vi "Win32 Decode Img Stream.vi"(8 "error in (no error)":errorcluster, 10 "Dest Format":string(combo)="{d98c6b95-3efe-47d6-bb25-eb1748ab0cf1}", 11 "Image Data":u8[](array[numeric])) -> (0 "error out":errorcluster, 1 "Image Height":u32, 2 "Image Width":u32, 3 "Dest":u32[][](array[numeric]), 4 "Image Stride":u32)   [LabVIEW 2020]
uses:
  ole32.dll
  windowscodecs.dll
  shlwapi.dll
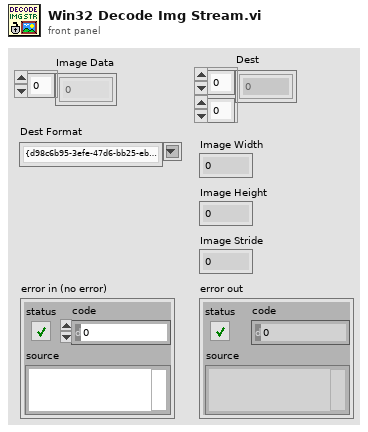
[diagram p1: front panel]
types:
  T1 = cluster{"GUID1":u32, "GUID2":u16, "GUID3":u16, "GUID4":cluster{"GUID4[0]":u8, "GUID4[1]":u8, "GUID4[2]":u8, "GUID4[3]":u8, "GUID4[4]":u8, "GUID4[5]":u8, "GUID4[6]":u8, "GUID4[7]":u8}}
  T2 = enum32{"Custom", "MedianCut", "FixedBW", "FixedHalftone8", "FixedHalftone27", "FixedHalftone64", "FixedHalftone125", "FixedHalftone216 / FixedWebPalette", "FixedHalftone252", "FixedHalftone256", "FixedGray4", "FixedGray16", "FixedGray256"}
  T3 = enum32{"None / Solid", "Ordered4x4", "Ordered8x8", "Ordered16x16", "Spiral4x4", "Spiral8x8", "DualSpiral4x4", "DualSpiral8x8", "ErrorDiffusion"}
  T4 = enum32{"NoCache", "CacheOnDemand", "CacheOnLoad"}
  T5 = cluster{"puiWidth":u32, "puiWidth":u32, "puiWidth":u32, "puiHeight":u32}
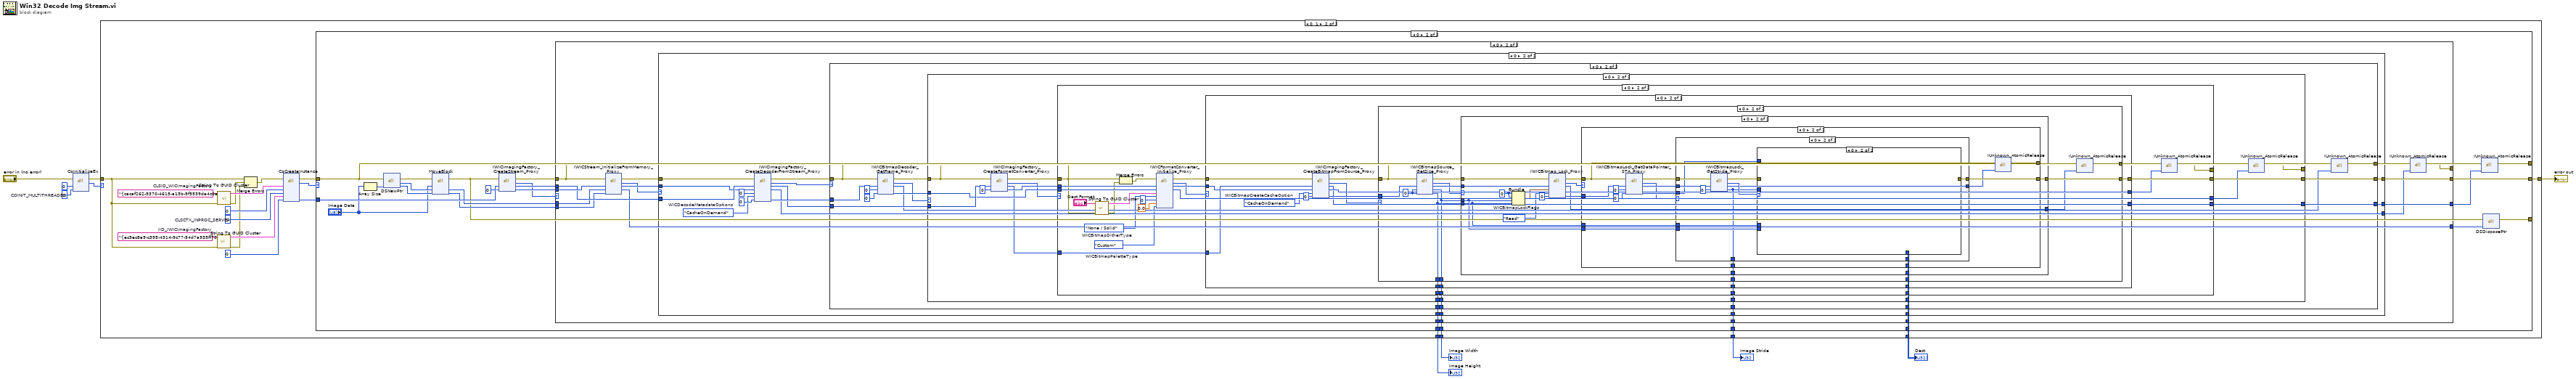
[diagram p0: block diagram]
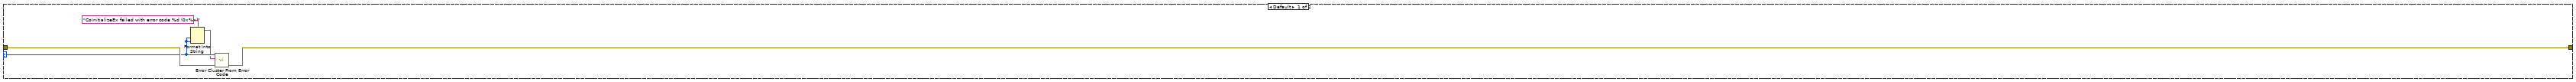
[diagram p2: hidden frame]
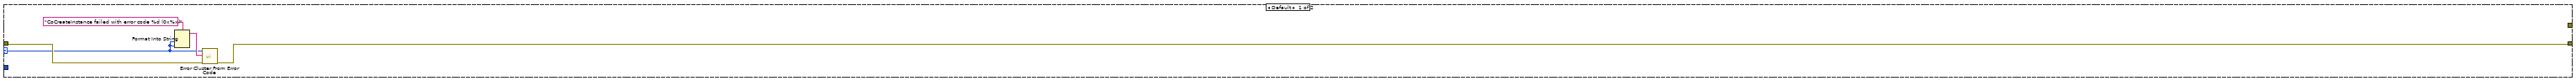
[diagram p3: hidden frame]
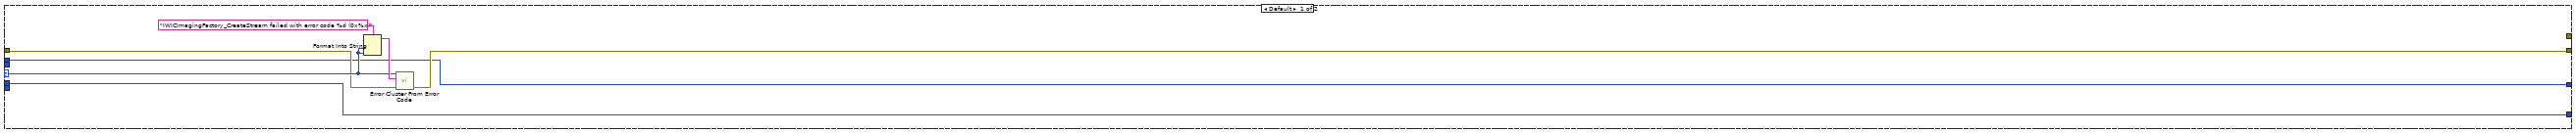
[diagram p4: hidden frame]
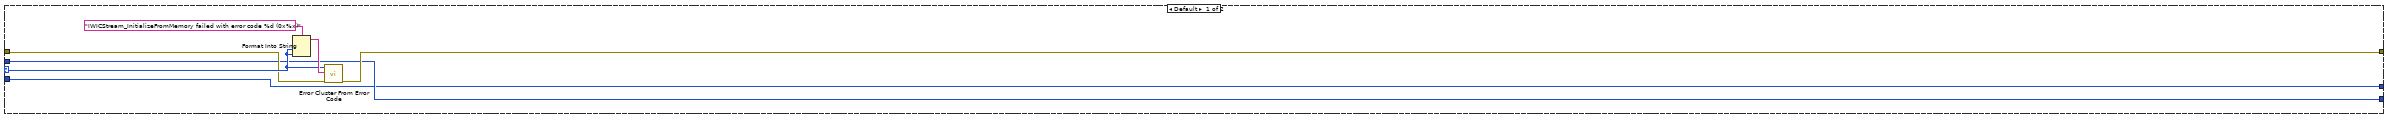
[diagram p5: hidden frame]
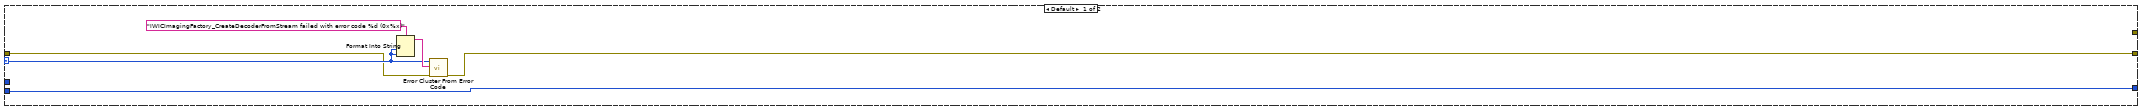
[diagram p6: hidden frame]
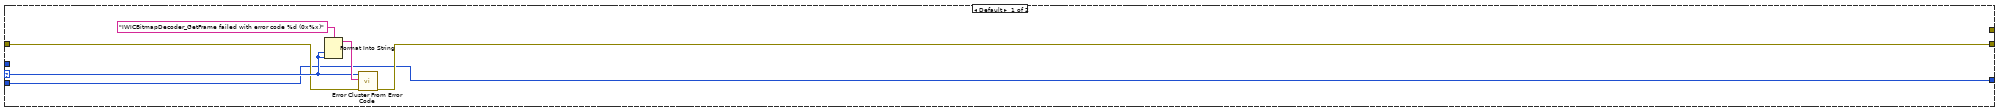
[diagram p7: hidden frame]
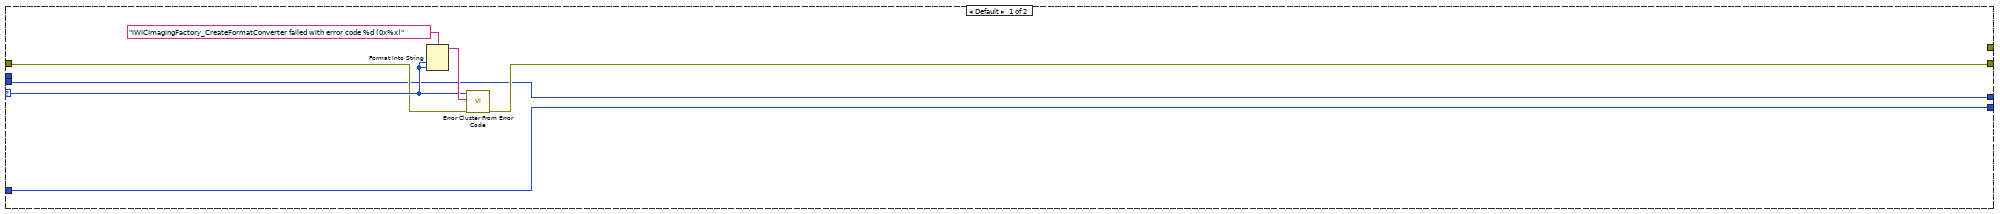
[diagram p8: hidden frame]
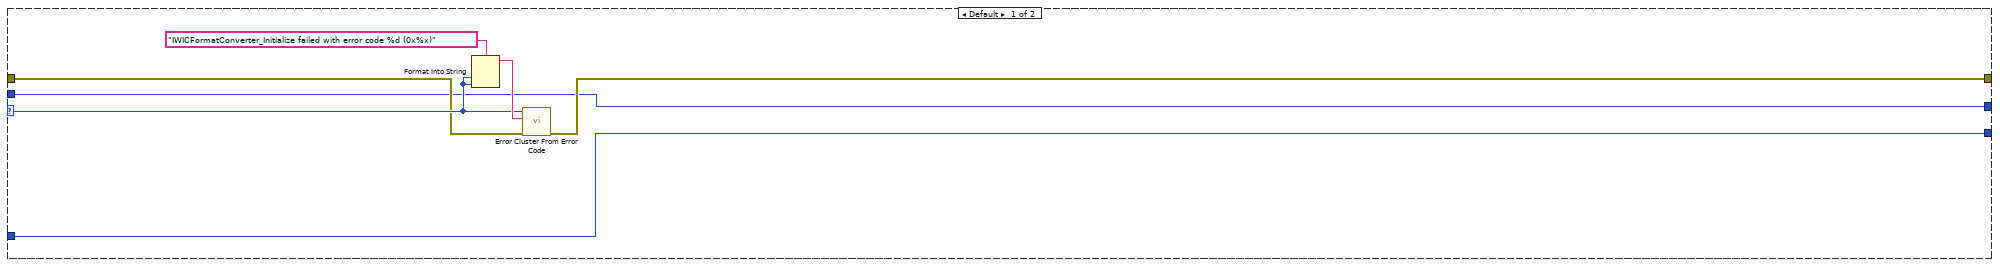
[diagram p9: hidden frame]
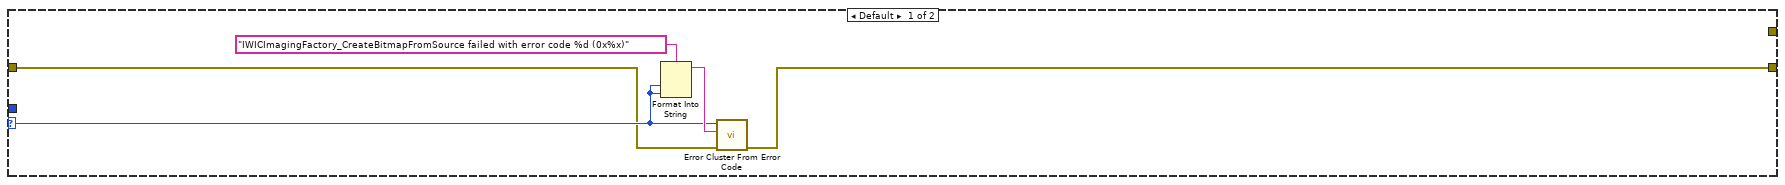
[diagram p10: hidden frame]
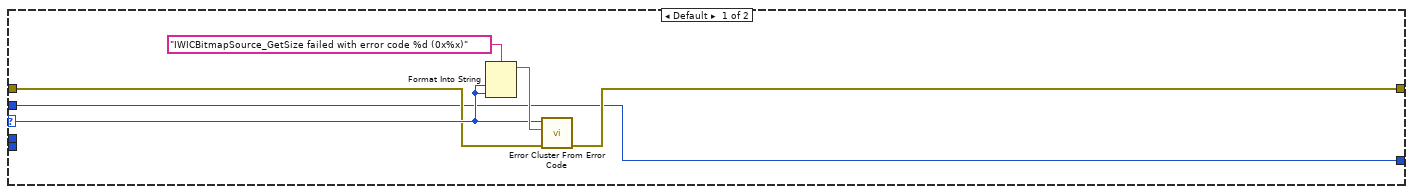
[diagram p11: hidden frame]
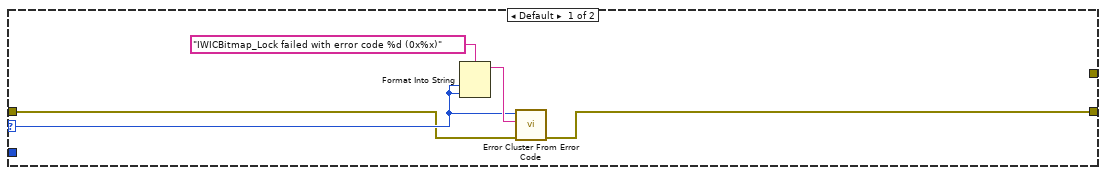
[diagram p12: hidden frame]
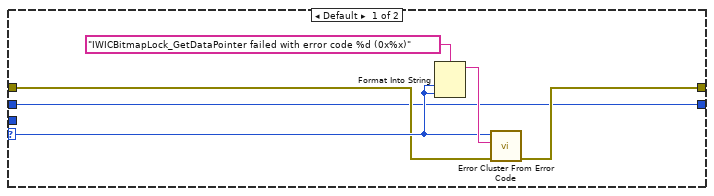
[diagram p13: hidden frame]
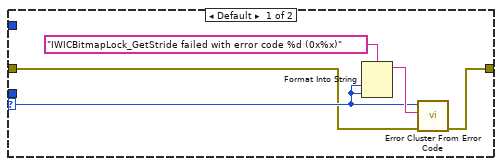
[diagram p14: hidden frame]
diagram:
  w9 = u32 0  # COINIT_MULTITHREADED
  n1 = dll-call lib="ole32.dll" fn="CoInitializeEx"(error in="error in (no error)", "pvReserved"=u64 0, "dwCoInit"=w9) -> (error out=w8:errorcluster, "Return"=w6:i32)  [unwired: 4 in, 1 out]
  n2 = case shown="0, 1" w6 {
    selector: w6 -> [w13 _]
    tunnel: w8 -> [w15 w25]
    tunnel: [w11 w20] -> w5
    tunnel: [_ w19] -> w4
    tunnel: [_ w18] -> w3
    tunnel: [_ w17] -> w2
    tunnel: [_ w16] -> w1
    frame Default {
      n3 = Format Into String(format string="CoInitializeEx failed with error code %d (0x%x)" ("error message (\"\")"), w13, w13) -> (resulting string=w12:string)  [unwired: 2 in, 1 out]
      n4 = call <vilib>:"Error Cluster From Error Code.vi"("error in (no error)"=w15, "error message (\"\")"=w12, "error code (0)"=w13) -> ("error out"=w11:errorcluster)  [unwired: 6 in]
    }
    frame 0, 1 {
      w30 = "{ec5ec8a9-c395-4314-9c77-54d7a935ff70}"  # IID_IWICImagingFactory
      w32 = u32 1  # CLSCTX_INPROC_SERVER
      w34 = "{cacaf262-9370-4615-a13b-9f5539da4c0a}"  # CLSID_WICImagingFactory
      n5 = call "String To GUID Cluster.vi"("error in (no error)"=w25, "Input String"=w30) -> ("error out"=w23:errorcluster, "GUID"=w29:T1)  [unwired: 4 in]
      n6 = call "String To GUID Cluster.vi"("error in (no error)"=w25, "Input String"=w34) -> ("error out"=w24:errorcluster, "GUID"=w33:T1)  [unwired: 4 in]
      n7 = Merge Errors(w25, w24, w23) -> (w22:errorcluster)
      n8 = dll-call lib="ole32.dll" fn="CoCreateInstance"(error in=w22, "rclsid"=w33, "pUnkOuter"=u64 0, "dwClsContext"=w32, "riid"=w29, "ppv"=u64 0) -> (error out=w27:errorcluster, "Return"=w21:i32, "ppv"=w26:u64)  [unwired: 6 in, 1 out]
      n9 = case shown="0" w21 {
        selector: w21 -> [w36 _]
        tunnel: w27 -> [w37 w42]
        tunnel: w26 -> [_ w63]
        tunnel: [w35 w58] -> w20
        tunnel: [_ w41] -> _
        tunnel: [_ w47] -> _
        tunnel: [_ w46] -> w19
        tunnel: [_ w45] -> w18
        tunnel: [_ w44] -> w17
        tunnel: [_ w43] -> w16
        frame Default {
          n10 = Format Into String(format string="CoCreateInstance failed with error code %d (0x%x)" ("error message (\"\")"), w36, w36) -> (resulting string=w38:string)  [unwired: 2 in, 1 out]
          n11 = call <vilib>:"Error Cluster From Error Code.vi"("error in (no error)"=w37, "error message (\"\")"=w38, "error code (0)"=w36) -> ("error out"=w35:errorcluster)  [unwired: 6 in]
        }
        frame 0 {
          n12 = Array Size(array="Image Data") -> (size(s)=w53:i32)
          n13 = dll-call lib="LabVIEW" fn="DSNewPtr"(error in=w42, "Size"=w53) -> (error out=w57:errorcluster, "Ptr"=w56:u64, "Size"=w55:i32)  [unwired: 2 in, 1 out]
          n14 = dll-call lib="LabVIEW" fn="MoveBlock"(error in=w57, "Src"="Image Data", "Dest"=w56, "Size"=w55) -> (error out=w48:errorcluster, "Dest"=w52:u64, "Size"=w51:i32)  [unwired: 4 in, 1 out]
          n15 = dll-call lib="windowscodecs.dll" fn="IWICImagingFactory_CreateStream_Proxy" label="IWICImagingFactory_CreateStream"(error in=w48, "IWICFactory"=w63, "ppIWICStream"=u64 0) -> (error out=w50:errorcluster, "Return"=w59:i32, "IWICFactory"=w60:u64, "ppIWICStream"=w61:u64)  [unwired: 2 in, 1 out]
          n16 = case shown="0" w59 {
            selector: w59 -> [w68 _]
            tunnel: w50 -> [w67 w73]
            tunnel: w61 -> [_ w87]
            tunnel: w60 -> [w64 w86]
            tunnel: [w66 w80] -> w58
            tunnel: w52 -> [w65 w82]
            tunnel: w51 -> [_ w81]
            tunnel: [_ w72] -> _
            tunnel: [w65 w79] -> w49
            tunnel: [w64 w78] -> w40
            tunnel: [_ w77] -> w46
            tunnel: [_ w76] -> w45
            tunnel: [_ w75] -> w44
            tunnel: [_ w74] -> w43
            frame Default {
              n17 = Format Into String(format string="IWICImagingFactory_CreateStream failed with error code %d (0x%x)" ("error message (\"\")"), w68, w68) -> (resulting string=w69:string)  [unwired: 2 in, 1 out]
              n18 = call <vilib>:"Error Cluster From Error Code.vi"("error in (no error)"=w67, "error message (\"\")"=w69, "error code (0)"=w68) -> ("error out"=w66:errorcluster)  [unwired: 6 in]
            }
            frame 0 {
              n19 = dll-call lib="windowscodecs.dll" fn="IWICStream_InitializeFromMemory_Proxy" label="IWICStream_InitializeFromMemory"(error in=w73, "IWICStream"=w87, "pbBuffer"=w82, "cbBufferSize"=w81) -> (error out=w83:errorcluster, "Return"=w84:i32, "IWICStream"=w85:u64, "pbBuffer"=w79:u64)  [unwired: 3 in, 1 out]
              n20 = case shown="0" w84 {
                selector: w84 -> [w92 _]
                tunnel: w83 -> [w91 w111]
                tunnel: w86 -> [w88 w110]
                tunnel: w85 -> [w89 w109]
                tunnel: [w90 w102] -> w80
                tunnel: [w89 w100] -> w71
                tunnel: [w88 w99] -> w78
                tunnel: [_ w98] -> w77
                tunnel: [_ w97] -> w76
                tunnel: [_ w96] -> w75
                tunnel: [_ w95] -> w74
                frame Default {
                  n21 = Format Into String(format string="IWICStream_InitializeFromMemory failed with error code %d (0x%x)" ("error message (\"\")"), w92, w92) -> (resulting string=w93:string)  [unwired: 2 in, 1 out]
                  n22 = call <vilib>:"Error Cluster From Error Code.vi"("error in (no error)"=w91, "error message (\"\")"=w93, "error code (0)"=w92) -> ("error out"=w90:errorcluster)  [unwired: 6 in]
                }
                frame 0 {
                  w104 = enum32{"CacheOnDemand", "CacheOnLoad"}."CacheOnDemand"  # WICDecodeMetadataOptions
                  n23 = dll-call lib="windowscodecs.dll" fn="IWICImagingFactory_CreateDecoderFromStream_Proxy" label="IWICImagingFactory_CreateDecoderFromStream"(error in=w111, "IWICFactory"=w110, "pIStream"=w109, "pguidVendor"=u64 0, "metadataOptions"=w104, "ppIDecoder"=u64 0) -> (error out=w101:errorcluster, "Return"=w103:i32, "IWICFactory"=w105:u64, "pIStream"=w100:u64, "ppIDecoder"=w106:u64)  [unwired: 4 in, 1 out]
                  n24 = case shown="0" w103 {
                    selector: w103 -> [w115 _]
                    tunnel: w101 -> [w114 w120]
                    tunnel: w106 -> [_ w133]
                    tunnel: w105 -> [w112 w130]
                    tunnel: [w113 w127] -> w102
                    tunnel: [_ w119] -> _
                    tunnel: [w112 w125] -> w99
                    tunnel: [_ w124] -> w98
                    tunnel: [_ w123] -> w97
                    tunnel: [_ w122] -> w96
                    tunnel: [_ w121] -> w95
                    frame Default {
                      n25 = Format Into String(format string="IWICImagingFactory_CreateDecoderFromStream failed with error code %d (0x%x)" ("error message (\"\")"), w115, w115) -> (resulting string=w116:string)  [unwired: 2 in, 1 out]
                      n26 = call <vilib>:"Error Cluster From Error Code.vi"("error in (no error)"=w114, "error message (\"\")"=w116, "error code (0)"=w115) -> ("error out"=w113:errorcluster)  [unwired: 6 in]
                    }
                    frame 0 {
                      n27 = dll-call lib="windowscodecs.dll" fn="IWICBitmapDecoder_GetFrame_Proxy" label="IWICBitmapDecoder_GetFrame"(error in=w120, "IWICBitmapDecoder"=w133, "index"=u32 0, "ppIBitmapFrame"=u64 0) -> (error out=w126:errorcluster, "Return"=w128:i32, "IWICBitmapDecoder"=w118:u64, "ppIBitmapFrame"=w129:u64)  [unwired: 3 in, 1 out]
                      n28 = case shown="0" w128 {
                        selector: w128 -> [w137 _]
                        tunnel: w126 -> [w136 w142]
                        tunnel: w130 -> [w134 w155]
                        tunnel: w129 -> [_ w152]
                        tunnel: [w135 w149] -> w127
                        tunnel: [_ w141] -> _
                        tunnel: [w134 w147] -> w125
                        tunnel: [_ w146] -> w124
                        tunnel: [_ w145] -> w123
                        tunnel: [_ w144] -> w122
                        tunnel: [_ w143] -> w121
                        frame Default {
                          n29 = Format Into String(format string="IWICBitmapDecoder_GetFrame failed with error code %d (0x%x)" ("error message (\"\")"), w137, w137) -> (resulting string=w138:string)  [unwired: 2 in, 1 out]
                          n30 = call <vilib>:"Error Cluster From Error Code.vi"("error in (no error)"=w136, "error message (\"\")"=w138, "error code (0)"=w137) -> ("error out"=w135:errorcluster)  [unwired: 6 in]
                        }
                        frame 0 {
                          n31 = dll-call lib="windowscodecs.dll" fn="IWICImagingFactory_CreateFormatConverter_Proxy" label="IWICImagingFactory_CreateFormatConverter"(error in=w142, "IWICFactory"=w155, "ppIFormatConverter"=u64 0) -> (error out=w148:errorcluster, "Return"=w150:i32, "IWICFactory"=w151:u64, "ppIFormatConverter"=w153:u64)  [unwired: 2 in, 1 out]
                          n32 = case shown="0" w150 {
                            selector: w150 -> [w160 _]
                            tunnel: w148 -> [w159 w165]
                            tunnel: w153 -> [_ w186]
                            tunnel: w152 -> [w157 w185]
                            tunnel: w151 -> [w156 w178]
                            tunnel: [w158 w175] -> w149
                            tunnel: [w157 w173] -> w140
                            tunnel: [_ w164] -> _
                            tunnel: [w156 w170] -> w147
                            tunnel: [_ w169] -> w146
                            tunnel: [_ w168] -> w145
                            tunnel: [_ w167] -> w144
                            tunnel: [_ w166] -> w143
                            frame Default {
                              n33 = Format Into String(format string="IWICImagingFactory_CreateFormatConverter failed with error code %d (0x%x)" ("error message (\"\")"), w160, w160) -> (resulting string=w161:string)  [unwired: 2 in, 1 out]
                              n34 = call <vilib>:"Error Cluster From Error Code.vi"("error in (no error)"=w159, "error message (\"\")"=w161, "error code (0)"=w160) -> ("error out"=w158:errorcluster)  [unwired: 6 in]
                            }
                            frame 0 {
                              w180 = T2."Custom"  # WICBitmapPaletteType
                              w183 = T3."None / Solid"  # WICBitmapDitherType
                              n35 = call "String To GUID Cluster.vi"("error in (no error)"=w165, "Input String"="Dest Format") -> ("error out"=w172:errorcluster, "GUID"=w184:T1)  [unwired: 4 in]
                              n36 = Merge Errors(w165, w172) -> (w171:errorcluster)
                              n37 = dll-call lib="windowscodecs.dll" fn="IWICFormatConverter_Initialize_Proxy" label="IWICFormatConverter_Initialize"(error in=w171, "IWICFormatConverter"=w186, "pISource"=w185, "dstFormat"=w184, "dither"=w183, "pIPalette"=u64 0, "alphaThresholdPercent"=0.0, "paletteTranslate"=w180) -> (error out=w174:errorcluster, "Return"=w176:i32, "IWICFormatConverter"=w177:u64, "pISource"=w173:u64)  [unwired: 7 in, 1 out]
                              n38 = case shown="0" w176 {
                                selector: w176 -> [w191 _]
                                tunnel: w174 -> [w190 w208]
                                tunnel: w178 -> [w187 w207]
                                tunnel: w177 -> [w188 w206]
                                tunnel: [w189 w201] -> w175
                                tunnel: [w188 w199] -> w163
                                tunnel: [w187 w198] -> w170
                                tunnel: [_ w197] -> w169
                                tunnel: [_ w196] -> w168
                                tunnel: [_ w195] -> w167
                                tunnel: [_ w194] -> w166
                                frame Default {
                                n39 = Format Into String(format string="IWICFormatConverter_Initialize failed with error code %d (0x%x)" ("error message (\"\")"), w191, w191) -> (resulting string=w192:string)  [unwired: 2 in, 1 out]
                                n40 = call <vilib>:"Error Cluster From Error Code.vi"("error in (no error)"=w190, "error message (\"\")"=w192, "error code (0)"=w191) -> ("error out"=w189:errorcluster)  [unwired: 6 in]
                                }
                                frame 0 {
                                w205 = T4."CacheOnDemand"  # WICBitmapCreateCacheOption
                                n41 = dll-call lib="windowscodecs.dll" fn="IWICImagingFactory_CreateBitmapFromSource_Proxy" label="IWICImagingFactory_CreateBitmapFromSource"(error in=w208, "IWICFactory"=w207, "pIBitmapSource"=w206, "option"=w205, "ppIBitmap"=u64 0) -> (error out=w200:errorcluster, "Return"=w202:i32, "IWICFactory"=w198:u64, "pIBitmapSource"=w199:u64, "ppIBitmap"=w203:u64)  [unwired: 3 in, 1 out]
                                n42 = case shown="0" w202 {
                                selector: w202 -> [w211 _]
                                tunnel: w200 -> [w210 w216]
                                tunnel: w203 -> [_ w226]
                                tunnel: [w209 w221] -> w201
                                tunnel: [_ w215] -> _
                                tunnel: [_ w220] -> w197
                                tunnel: [_ w219] -> w196
                                tunnel: [_ w218] -> w195
                                tunnel: [_ w217] -> w194
                                frame Default {
                                n43 = Format Into String(format string="IWICImagingFactory_CreateBitmapFromSource failed with error code %d (0x%x)" ("error message (\"\")"), w211, w211) -> (resulting string=w212:string)  [unwired: 2 in, 1 out]
                                n44 = call <vilib>:"Error Cluster From Error Code.vi"("error in (no error)"=w210, "error message (\"\")"=w212, "error code (0)"=w211) -> ("error out"=w209:errorcluster)  [unwired: 6 in]
                                }
                                frame 0 {
                                w225 = u32 0 ("puiWidth")
                                n45 = dll-call lib="windowscodecs.dll" fn="IWICBitmapSource_GetSize_Proxy" label="IWICBitmapSource_GetSize"(error in=w216, "IWICBitmapSource"=w226, "puiWidth"=w225, "puiHeight"=w225) -> (error out=w224:errorcluster, "Return"=w222:i32, "IWICBitmapSource"=w223:u64, "puiWidth"=w218:u32, "puiHeight"=w217:u32)  [unwired: 2 in, 1 out]
                                n46 = case shown="0" w222 {
                                selector: w222 -> [w230 _]
                                tunnel: w224 -> [w229 w246]
                                tunnel: w223 -> [w227 w245]
                                tunnel: w218 -> [_ w241]
                                tunnel: w217 -> [_ w240]
                                tunnel: [w228 w238] -> w221
                                tunnel: [w227 w235] -> w214
                                tunnel: [_ w234] -> w220
                                tunnel: [_ w233] -> w219
                                frame Default {
                                n47 = Format Into String(format string="IWICBitmapSource_GetSize failed with error code %d (0x%x)" ("error message (\"\")"), w230, w230) -> (resulting string=w231:string)  [unwired: 2 in, 1 out]
                                n48 = call <vilib>:"Error Cluster From Error Code.vi"("error in (no error)"=w229, "error message (\"\")"=w231, "error code (0)"=w230) -> ("error out"=w228:errorcluster)  [unwired: 6 in]
                                }
                                frame 0 {
                                w243 = enum32{"None", "Read", "Write"}."Read"  # WICBitmapLockFlags
                                w247 = u32 0 ("puiWidth")
                                n49 = Bundle("puiWidth"=w247, "puiWidth"=w247, "puiWidth"=w241, "puiHeight"=w240) -> (w244:T5)  [unwired: 1 in]
                                n50 = dll-call lib="windowscodecs.dll" fn="IWICBitmap_Lock_Proxy" label="IWICBitmap_Lock"(error in=w246, "IWICBitmapSource"=w245, "prcLock"=w244, "flags"=w243, "ppILock"=u64 0) -> (error out=w236:errorcluster, "Return"=w239:i32, "IWICBitmapSource"=w235:u64, "ppILock"=w237:u64)  [unwired: 4 in, 1 out]
                                n51 = case shown="0" w239 {
                                selector: w239 -> [w250 _]
                                tunnel: w236 -> [w249 w256]
                                tunnel: w237 -> [_ w267]
                                tunnel: w241 -> [_ w261]
                                tunnel: w240 -> [_ w260]
                                tunnel: [w248 w258] -> w238
                                tunnel: [_ w255] -> _
                                tunnel: [_ w254] -> w234
                                tunnel: [_ w253] -> w233
                                frame Default {
                                n52 = Format Into String(format string="IWICBitmap_Lock failed with error code %d (0x%x)" ("error message (\"\")"), w250, w250) -> (resulting string=w251:string)  [unwired: 2 in, 1 out]
                                n53 = call <vilib>:"Error Cluster From Error Code.vi"("error in (no error)"=w249, "error message (\"\")"=w251, "error code (0)"=w250) -> ("error out"=w248:errorcluster)  [unwired: 6 in]
                                }
                                frame 0 {
                                n54 = dll-call lib="windowscodecs.dll" fn="IWICBitmapLock_GetDataPointer_STA_Proxy" label="IWICBitmapLock_GetDataPointer"(error in=w256, "IWICBitmapLock"=w267, "pcbBufferSize"=u32 0, "ppbData"=u64 0) -> (error out=w264:errorcluster, "Return"=w259:i32, "IWICBitmapLock"=w263:u64, "ppbData"=w262:u64)  [unwired: 3 in, 1 out]
                                n55 = case shown="0" w259 {
                                selector: w259 -> [w271 _]
                                tunnel: w264 -> [w270 w285]
                                tunnel: w263 -> [w268 w284]
                                tunnel: w262 -> [_ w281]
                                tunnel: w261 -> [_ w280]
                                tunnel: w260 -> [_ w279]
                                tunnel: [w269 w277] -> w258
                                tunnel: [w268 w276] -> w257
                                tunnel: [_ w275] -> w254
                                tunnel: [_ w274] -> w253
                                frame Default {
                                n56 = Format Into String(format string="IWICBitmapLock_GetDataPointer failed with error code %d (0x%x)" ("error message (\"\")"), w271, w271) -> (resulting string=w272:string)  [unwired: 2 in, 1 out]
                                n57 = call <vilib>:"Error Cluster From Error Code.vi"("error in (no error)"=w270, "error message (\"\")"=w272, "error code (0)"=w271) -> ("error out"=w269:errorcluster)  [unwired: 6 in]
                                }
                                frame 0 {
                                n58 = dll-call lib="windowscodecs.dll" fn="IWICBitmapLock_GetStride_Proxy" label="IWICBitmapLock_GetStride"(error in=w285, "IWICBitmapLock"=w284, "pcbStride"=u32 0) -> (error out=w282:errorcluster, "Return"=w278:i32, "IWICBitmapLock"=w276:u64, "pcbStride"=w274:u32)  [unwired: 2 in, 1 out]
                                n59 = case shown="0" w278 {
                                selector: w278 -> [w288 _]
                                tunnel: w282 -> [w287 w299]
                                tunnel: w281 -> [_ w297]
                                tunnel: w274 -> [_ w295]
                                tunnel: w280 -> [_ w294]
                                tunnel: w279 -> [_ w293]
                                tunnel: [w286 w292] -> w277
                                tunnel: [_ w291] -> w275
                                frame Default {
                                n60 = Format Into String(format string="IWICBitmapLock_GetStride failed with error code %d (0x%x)" ("error message (\"\")"), w288, w288) -> (resulting string=w290:string)  [unwired: 2 in, 1 out]
                                n61 = call <vilib>:"Error Cluster From Error Code.vi"("error in (no error)"=w287, "error message (\"\")"=w290, "error code (0)"=w288) -> ("error out"=w286:errorcluster)  [unwired: 6 in]
                                }
                                frame 0 {
                                w300 = u32 0  # U32
                                # "We get 32-bit RGB 2D array here. Change the representation\nand MoveBlock params if you need other image type."
                                n62 = Compound Arithmetic op=MULTIPLY(w295, w293) -> (w296:u32)
                                n63 = Initialize Array(w300, w293, w294) -> (w298:u32[][])
                                n64 = dll-call lib="LabVIEW" fn="MoveBlock"(error in=w299, "Src"=w297, "Dest"=w298, "Size"=w296) -> (error out=w292:errorcluster, "Dest"=w291:u32[][])  [unwired: 5 in, 1 out]
                                }
                                }
                                }
                                }
                                n65 = dll-call lib="shlwapi.dll" fn="IUnknown_AtomicRelease"(error in=w256, "ppunk"=w257) -> (error out=w255:errorcluster)  [unwired: 4 in, 1 out]
                                }
                                }
                                }
                                }
                                n66 = dll-call lib="shlwapi.dll" fn="IUnknown_AtomicRelease"(error in=w216, "ppunk"=w214) -> (error out=w215:errorcluster)  [unwired: 4 in, 1 out]
                                }
                                }
                                }
                              }
                              n67 = dll-call lib="shlwapi.dll" fn="IUnknown_AtomicRelease"(error in=w165, "ppunk"=w163) -> (error out=w164:errorcluster)  [unwired: 4 in, 1 out]
                            }
                          }
                          n68 = dll-call lib="shlwapi.dll" fn="IUnknown_AtomicRelease"(error in=w142, "ppunk"=w140) -> (error out=w141:errorcluster)  [unwired: 4 in, 1 out]
                        }
                      }
                      n69 = dll-call lib="shlwapi.dll" fn="IUnknown_AtomicRelease"(error in=w120, "ppunk"=w118) -> (error out=w119:errorcluster)  [unwired: 4 in, 1 out]
                    }
                  }
                }
              }
              n70 = dll-call lib="shlwapi.dll" fn="IUnknown_AtomicRelease"(error in=w73, "ppunk"=w71) -> (error out=w72:errorcluster)  [unwired: 4 in, 1 out]
            }
          }
          n71 = dll-call lib="shlwapi.dll" fn="IUnknown_AtomicRelease"(error in=w42, "ppunk"=w40) -> (error out=w41:errorcluster)  [unwired: 4 in, 1 out]
          n72 = dll-call lib="LabVIEW" fn="DSDisposePtr"(error in=w48, "Ptr"=w49) -> (error out=w47:errorcluster)  [unwired: 4 in, 1 out]
        }
      }
    }
  }
  "error out" <- w5
  "Image Width" <- w2
  "Image Height" <- w1
  "Image Stride" <- w3
  "Dest" <- w4
